vi "Set Message Broker.vi"(8 "error in (no error)":errorcluster, 10 "Broker":refnum<data-value>, 11 "Message Broker Interface Ref in":refnum<class "Message Broker Interface Ref.lvclass">) -> (0 "error out":errorcluster, 3 "Message Broker Interface Ref out":refnum<class "Message Broker Interface Ref.lvclass">)   [LabVIEW 2016, in "Stream Mediator.lvlib" / "Message Broker Interface Ref.lvclass"]
doc: "--\nCopyright © 2017 Composed SystemsI All rights reserved.\n\nAuthor: Jon McBee <jon.mcbee@composed.io>\n\nThis library is provided \"AS IS\" ,WITHOUT WARRANTIES OR\nCONDITIONS OF ANY KIND, either express or implied.\n\nComposed Systems -- composed.io\n\nStream 0.0.1.1\nJon McBee - Composed Systems\nCopyright (c) 2017, Composed Systems"
uses:
  <userlib>/Composed Systems/Stream/Mediator/Classes/Message Broker Interface Ref/Message Broker Interface Ref.lvclass
  <userlib>/Composed Systems/Stream/Mediator/Classes/Message Broker/Message Broker.lvclass
  <userlib>/Composed Systems/Stream/Mediator/Classes/Message Broker Interface Ref/Message Broker Interface Ref.lvclass/Message Broker Interface Ref.ctl
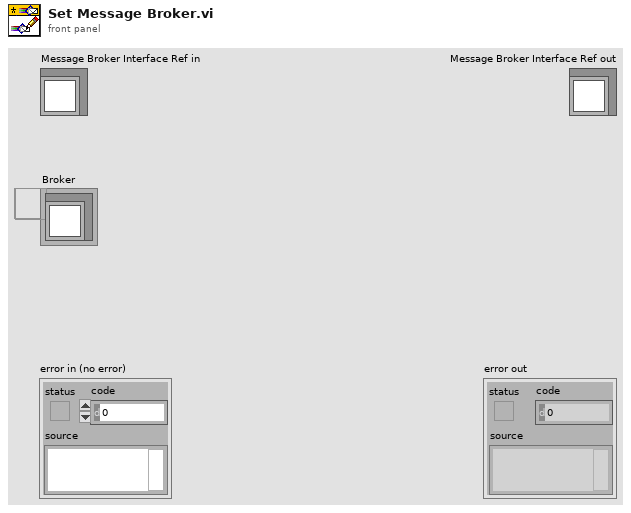
[diagram p1: front panel]
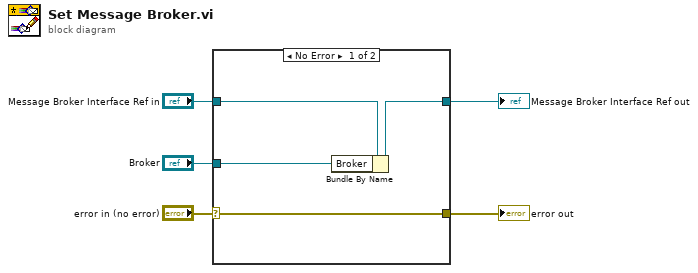
[diagram p0: block diagram]
diagram:
  n1 = case shown="No Error" "error in (no error)" {
    selector: "error in (no error)" -> [w9 w11]
    tunnel: [w9 w11] -> w4
    tunnel: [w7 w10] -> w2
    tunnel: "Message Broker Interface Ref in" -> [w8 w10]
    tunnel: "Broker" -> [w6 _]
    frame No Error {
      n2 = Bundle By Name(cluster=w8, "Broker"=w6) -> (w7:refnum<class "Message Broker Interface Ref.lvclass">)
    }
    frame Error {
    }
  }
  "error out" <- w4
  "Message Broker Interface Ref out" <- w2
